vi "SetSettings.vi"(8 "error in (no error)":errorcluster, 10 "Settings":T1, 11 "configuration file path":path) -> (0 "error out":errorcluster)   [LabVIEW 2013]
uses:
  TypeDef/Settings.ctl
  <vilib>/Utility/config.llb/Write Key (String).vi
  <vilib>/Utility/config.llb/NI_LVConfig.lvlib
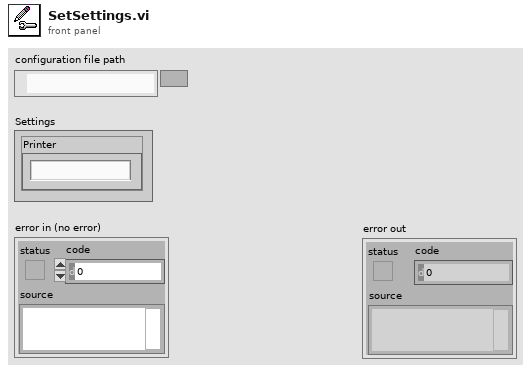
[diagram p1: front panel]
types:
  T1 = typedef "Settings.ctl" = cluster{"Printer":string}
  T2 = typedef "NI_LVConfig.lvlib/Config Data RefNum.ctl" = refnum<k1>
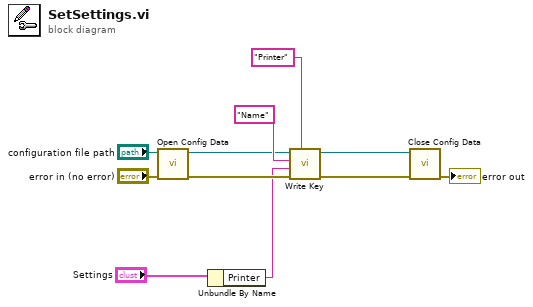
[diagram p0: block diagram]
diagram:
  n1 = call <vilib>:"Open Config Data.vi"("error in (no error)"="error in (no error)", "configuration file path"="configuration file path") -> ("error out"=w9:errorcluster, "refnum"=w8:T2)  [unwired: 7 in, 1 out]
  n2 = Unbundle By Name("Settings") -> ("Printer"=w1:string)
  n3 = call-poly <vilib>:"Write Key.vi"("section"="Printer", "error in (no error)"=w9, "value"=w1, "key"="Name", "refnum"=w8) -> ("error out"=w6:errorcluster, "refnum out"=w7:T2)  [unwired: 4 in, 1 out]
  n4 = call <vilib>:"Close Config Data.vi"("error in (no error)"=w6, "refnum"=w7) -> ("error out"=→"error out":errorcluster)  [unwired: 8 in, 1 out]
